vi "FTW-Client-Worker.vi"(1 "Shutdown Notification":refnum<notifier>, 2 "Endpoint Type":refnum<class "FTW-Endpoint.lvclass">, 3 "Address":string, 4 "Pipe":refnum<class "FTW-Endpoint.lvclass">) -> ()   [LabVIEW 2013, in "FTW-Client.lvclass"]
uses:
  FTW-Client.lvclass
  Endpoint/FTW-Endpoint.lvclass
panel:
  out "connected":bool
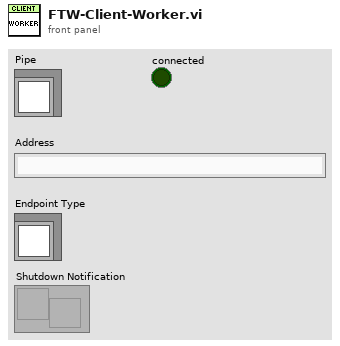
[diagram p1: front panel]
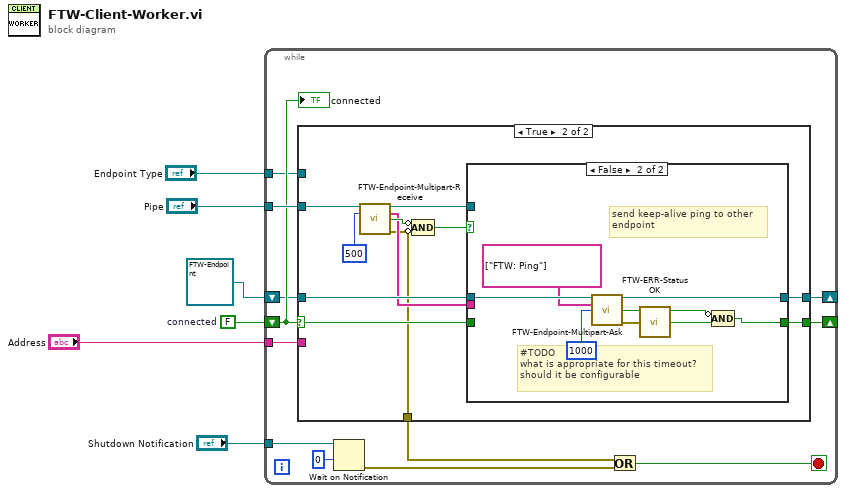
[diagram p0: block diagram]
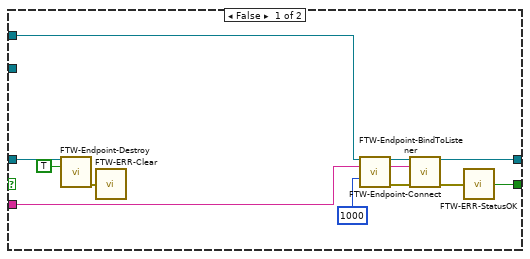
[diagram p2: hidden frame]
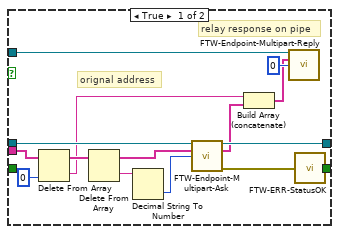
[diagram p3: hidden frame]
diagram:
  w5 = FALSE  # connected
  n1 = while {
    tunnel: "Pipe" -> [w18]
    shift-right: [w14] -> _
    shift-left: w5 -> [w17]
    shift-right: [w15] -> _
    shift-left: refnum<class "FTW-Endpoint.lvclass"> refnum ("FTW Endpoint") -> [w10]
    tunnel: "Address" -> [w16]
    tunnel: "Shutdown Notification" -> [w12]
    tunnel: "Endpoint Type" -> [w7]
    stop <- w9 stop-if-true
    n2 = case shown="True" w17 {
      selector: w17 -> [_ w33]
      tunnel: w18 -> [_ w41]
      tunnel: w16 -> [w27 _]
      tunnel: [w26 w38] -> w15
      tunnel: [w25 w34] -> w14
      tunnel: w10 -> [w22 w39]
      tunnel: [_ w31] -> w8
      tunnel: w7 -> [w19 _]
      frame False {
        n3 = call-dynamic "FTW-Endpoint-Destroy.vi"("FTW Endpoint"=w22, "Force Destroy"=TRUE) -> ("error out"=w20:errorcluster)  [unwired: 13 in]
        n4 = call "FTW-ERR-Clear.vi"("error to snuff"=w20) -> ()  [unwired: 1 out]
        n5 = call-dynamic "FTW-Endpoint-BindToListener.vi"("FTW-Endpoint In"=w19, "Address"=w27, "Timeout"=1000) -> ("FTW-Endpoint Out"=w30:refnum<class "FTW-Endpoint.lvclass">, "Actual Address"=w28:string, "error out"=w29:errorcluster)  [unwired: 10 in]
        n6 = call-dynamic "FTW-Endpoint-Connect.vi"("FTW Endpoint"=w30, "Endpoint Address"=w28, "error in"=w29) -> ("FTW Endpoint out"=w26:refnum<class "FTW-Endpoint.lvclass">, "error out"=w24:errorcluster)  [unwired: 11 in]
        n7 = call "FTW-ERR-StatusOK.vi"("error to check"=w24) -> ("Status OK?"=w25:bool)
      }
      frame True {
        n8 = call-dynamic "FTW-Endpoint-Multipart-Receive.vi"("FTW Endpoint"=w41, "Timeout"=500) -> ("FTW Endpoint out"=w35:refnum<class "FTW-Endpoint.lvclass">, "Message Received"=w32:string[], "Timed out?"=w37:bool, "error out"=w31:errorcluster)  [unwired: 10 in]
        n9 = Compound Arithmetic op=AND(invert w37, invert w31) -> (w36:bool)
        n10 = case shown="False" w36 {
          tunnel: w39 -> [w56 w64]
          tunnel: [w55 w63] -> w38
          tunnel: w32 -> [w45 _]
          tunnel: [w53 w58] -> w34
          tunnel: w35 -> [w52 _]
          tunnel: w33 -> [_ _]
          frame True {
            # "orignal address"
            # "relay response on pipe"
            n11 = Delete From Array(array=w45, index=0) -> (deleted portion=w42:string, array with subset deleted=w44:string[])  [unwired: 1 in]
            n12 = Delete From Array(array=w44) -> (deleted portion=w48:string, array with subset deleted=w49:string[])  [unwired: 2 in]
            n13 = Decimal String To Number(string=w48) -> (number=w47:i32)  [unwired: 2 in, 1 out]
            n14 = call-dynamic "FTW-Endpoint-Multipart-Ask.vi"("FTW Endpoint"=w56, "Multipart Message"=w49, "Read Timeout"=w47) -> ("FTW Endpoint out"=w55:refnum<class "FTW-Endpoint.lvclass">, "Reply"=w51:string[], "error out"=w54:errorcluster)  [unwired: 8 in, 2 out]
            n15 = Build Array (concatenate)(w42, w51) -> (w46:string[])
            n16 = call-dynamic "FTW-Endpoint-Multipart-Reply.vi"("FTW Endpoint"=w52, "Multipart Message"=w46, "Timeout"=0) -> ()  [unwired: 10 in, 3 out]
            n17 = call "FTW-ERR-StatusOK.vi"("error to check"=w54) -> ("Status OK?"=w53:bool)
          }
          frame False {
            # "send keep-alive ping to other\nendpoint"
            # "#TODO\nwhat is appropriate for this timeout?\nshould it be configurable"
            n18 = call-dynamic "FTW-Endpoint-Multipart-Ask.vi"("FTW Endpoint"=w64, "Multipart Message"=string[] ["FTW: Ping"], "Read Timeout"=1000) -> ("FTW Endpoint out"=w63:refnum<class "FTW-Endpoint.lvclass">, "Read Timed out?"=w57:bool, "error out"=w62:errorcluster)  [unwired: 8 in, 2 out]
            n19 = call "FTW-ERR-StatusOK.vi"("error to check"=w62) -> ("Status OK?"=w61:bool)
            n20 = Compound Arithmetic op=AND(invert w57, w61) -> (w58:bool)
          }
        }
      }
    }
    n21 = Wait on Notification(notifier=w12, timeout in ms (-1)=0) -> (error out=w11:errorcluster)  [unwired: 2 in, 3 out]
    n22 = Or(x=w8, y=w11) -> (x .or. y?=w9:bool)
    "connected" <- w17
  }
